vi "Apply Box.vi"(5 "Reading":string[](array[string])) -> (0 "Modes":cluster{"A=":u16, "B=":u16, "C=":u16, "D=":u16} {"D=" items=["T0+", "A+", "B+", "C+"]; "C=" items=["T0+", "A+", "B+", "D+"]; "B=" items=["T0+", "A+", "C+", "D+"]; "A=" items=["T0+", "B+", "C+", "D+"]}, 2 "Delays (s)":dbl[](array[numeric]) min=0.0 max=1000.0 format="%#_15f")   [LabVIEW 2009]
uses:
  <vilib>/regexp/Match Regular Expression.xnode
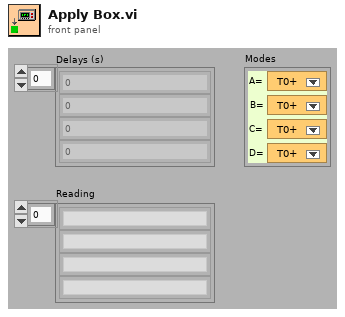
[diagram p1: front panel]
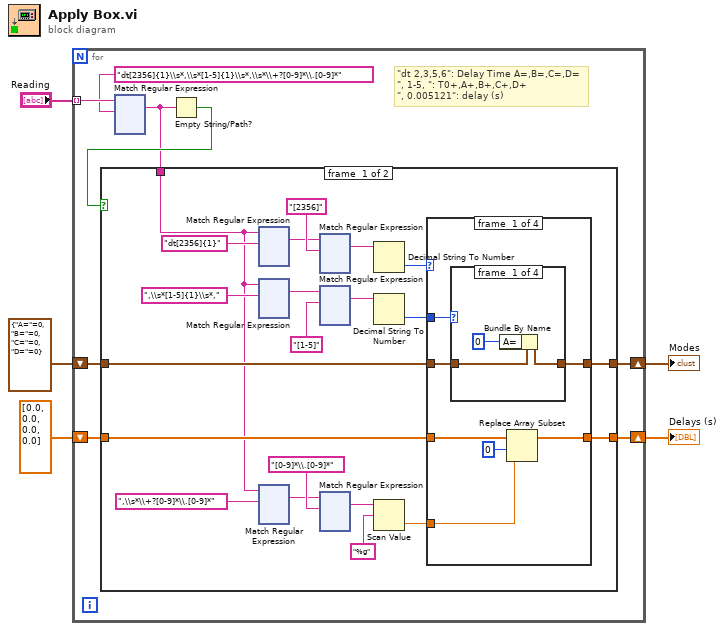
[diagram p0: block diagram]
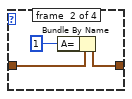
[diagram p2: hidden frame]
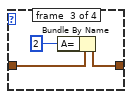
[diagram p3: hidden frame]
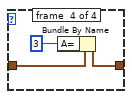
[diagram p4: hidden frame]
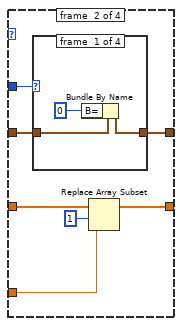
[diagram p5: hidden frame]
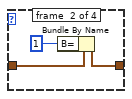
[diagram p6: hidden frame]
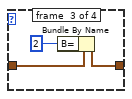
[diagram p7: hidden frame]
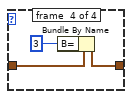
[diagram p8: hidden frame]
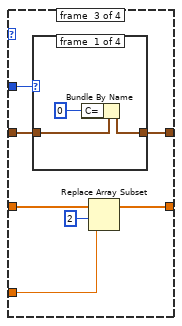
[diagram p9: hidden frame]
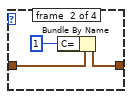
[diagram p10: hidden frame]
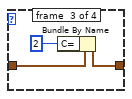
[diagram p11: hidden frame]
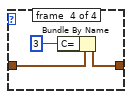
[diagram p12: hidden frame]
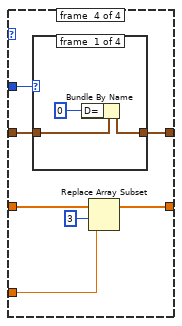
[diagram p13: hidden frame]
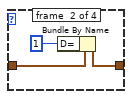
[diagram p14: hidden frame]
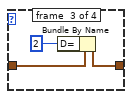
[diagram p15: hidden frame]
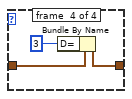
[diagram p16: hidden frame]
diagram:
  n1 = for {
    tunnel: "Reading" -> [w13] mode=indexing
    shift-right: [w6] -> w1
    shift-left: cluster{"A=":u16, "B=":u16, "C=":u16, "D=":u16} {"A="=0, "B="=0, "C="=0, "D="=0} ("Modes") -> [w9]
    shift-right: [w7] -> w2
    shift-left: dbl[] [0.0, 0.0, 0.0, 0.0] -> [w8]
    # "\"dt 2,3,5,6\": Delay Time A=,B=,C=,D=\n\", 1-5, \": T0+,A+,B+,C+,D+\n\", 0.005121\": delay (s)"
    n2 = xnode "Match Regular Expression"("input string"=w13, "regular expression"="dt[2356]{1}\\s*,\\s*[1-5]{1}\\s*,\\s*\\+?[0-9]*\\.[0-9]*") -> ("whole match"=w10:string)  [unwired: 4 in, 4 out]
    n3 = Empty String/Path?(string/path=w10) -> (empty?=w11:bool)
    n4 = case shown="False" w11 {
      tunnel: w10 -> [w17 _]
      tunnel: w9 -> [w22 w754]
      tunnel: w8 -> [w20 w753]
      tunnel: [w19 w753] -> w7
      tunnel: [w18 w754] -> w6
      frame #0 {
        n5 = xnode "Match Regular Expression"("input string"=w17, "regular expression"="dt[2356]{1}") -> ("whole match"=w16:string)  [unwired: 4 in, 4 out]
        n6 = xnode "Match Regular Expression"("input string"=w17, "regular expression"=",\\s*[1-5]{1}\\s*,") -> ("whole match"=w15:string)  [unwired: 4 in, 4 out]
        n7 = xnode "Match Regular Expression"("input string"=w17, "regular expression"=",\\s*\\+?[0-9]*\\.[0-9]*") -> ("whole match"=w14:string)  [unwired: 4 in, 4 out]
        n8 = xnode "Match Regular Expression"("input string"=w16, "regular expression"="[2356]") -> ("whole match"=w26:string)  [unwired: 4 in, 4 out]
        n9 = xnode "Match Regular Expression"("input string"=w15, "regular expression"="[1-5]") -> ("whole match"=w25:string)  [unwired: 4 in, 4 out]
        n10 = xnode "Match Regular Expression"("input string"=w14, "regular expression"="[0-9]*\\.[0-9]*") -> ("whole match"=w28:string)  [unwired: 4 in, 4 out]
        n11 = Decimal String To Number(string=w26) -> (number=w24:i32)  [unwired: 2 in, 1 out]
        n12 = Decimal String To Number(string=w25) -> (number=w23:i32)  [unwired: 2 in, 1 out]
        n13 = Scan Value(string=w28, format string="%g") -> (value=w21:dbl)  [unwired: 1 in, 1 out]
        n14 = case shown="2, Default" w24 {
          tunnel: w23 -> [w35 w54 w73 w92]
          tunnel: w22 -> [w41 w60 w79 w98]
          tunnel: w21 -> [w36 w55 w74 w93]
          tunnel: w20 -> [w39 w58 w77 w96]
          tunnel: [w38 w57 w76 w95] -> w19
          tunnel: [w40 w59 w78 w97] -> w18
          frame #0 {
            n15 = case shown="1, Default" w35 {
              tunnel: w41 -> [w43 w46 w49 w52]
              tunnel: [w42 w45 w48 w51] -> w40
              frame #0 {
                n16 = Bundle By Name(cluster=w43, "A="=u16 0) -> (w42:cluster{"A=":u16, "B=":u16, "C=":u16, "D=":u16})
              }
              frame #1 {
                n17 = Bundle By Name(cluster=w46, "A="=u16 1) -> (w45:cluster{"A=":u16, "B=":u16, "C=":u16, "D=":u16})
              }
              frame #2 {
                n18 = Bundle By Name(cluster=w49, "A="=u16 2) -> (w48:cluster{"A=":u16, "B=":u16, "C=":u16, "D=":u16})
              }
              frame #3 {
                n19 = Bundle By Name(cluster=w52, "A="=u16 3) -> (w51:cluster{"A=":u16, "B=":u16, "C=":u16, "D=":u16})
              }
            }
            n20 = Replace Array Subset(array=w39, new element=w36, index=0) -> (w38:dbl[])
          }
          frame #1 {
            n21 = case shown="1, Default" w54 {
              tunnel: w60 -> [w62 w65 w68 w71]
              tunnel: [w61 w64 w67 w70] -> w59
              frame #0 {
                n22 = Bundle By Name(cluster=w62, "B="=u16 0 ("A=")) -> (w61:cluster{"A=":u16, "B=":u16, "C=":u16, "D=":u16})
              }
              frame #1 {
                n23 = Bundle By Name(cluster=w65, "B="=u16 1 ("A=")) -> (w64:cluster{"A=":u16, "B=":u16, "C=":u16, "D=":u16})
              }
              frame #2 {
                n24 = Bundle By Name(cluster=w68, "B="=u16 2 ("A=")) -> (w67:cluster{"A=":u16, "B=":u16, "C=":u16, "D=":u16})
              }
              frame #3 {
                n25 = Bundle By Name(cluster=w71, "B="=u16 3 ("A=")) -> (w70:cluster{"A=":u16, "B=":u16, "C=":u16, "D=":u16})
              }
            }
            n26 = Replace Array Subset(array=w58, new element=w55, index=1) -> (w57:dbl[])
          }
          frame #2 {
            n27 = case shown="1, Default" w73 {
              tunnel: w79 -> [w81 w84 w87 w90]
              tunnel: [w80 w83 w86 w89] -> w78
              frame #0 {
                n28 = Bundle By Name(cluster=w81, "C="=u16 0 ("A=")) -> (w80:cluster{"A=":u16, "B=":u16, "C=":u16, "D=":u16})
              }
              frame #1 {
                n29 = Bundle By Name(cluster=w84, "C="=u16 1 ("A=")) -> (w83:cluster{"A=":u16, "B=":u16, "C=":u16, "D=":u16})
              }
              frame #2 {
                n30 = Bundle By Name(cluster=w87, "C="=u16 2 ("A=")) -> (w86:cluster{"A=":u16, "B=":u16, "C=":u16, "D=":u16})
              }
              frame #3 {
                n31 = Bundle By Name(cluster=w90, "C="=u16 3 ("A=")) -> (w89:cluster{"A=":u16, "B=":u16, "C=":u16, "D=":u16})
              }
            }
            n32 = Replace Array Subset(array=w77, new element=w74, index=2) -> (w76:dbl[])
          }
          frame #3 {
            n33 = case shown="1, Default" w92 {
              tunnel: w98 -> [w100 w103 w106 w109]
              tunnel: [w99 w102 w105 w108] -> w97
              frame #0 {
                n34 = Bundle By Name(cluster=w100, "D="=u16 0 ("A=")) -> (w99:cluster{"A=":u16, "B=":u16, "C=":u16, "D=":u16})
              }
              frame #1 {
                n35 = Bundle By Name(cluster=w103, "D="=u16 1 ("A=")) -> (w102:cluster{"A=":u16, "B=":u16, "C=":u16, "D=":u16})
              }
              frame #2 {
                n36 = Bundle By Name(cluster=w106, "D="=u16 2 ("A=")) -> (w105:cluster{"A=":u16, "B=":u16, "C=":u16, "D=":u16})
              }
              frame #3 {
                n37 = Bundle By Name(cluster=w109, "D="=u16 3 ("A=")) -> (w108:cluster{"A=":u16, "B=":u16, "C=":u16, "D=":u16})
              }
            }
            n38 = Replace Array Subset(array=w96, new element=w93, index=3) -> (w95:dbl[])
          }
        }
      }
      frame #1 {
      }
    }
  }
  "Modes" <- w1
  "Delays (s)" <- w2
